vi "Set Default Word.vi"(8 "error in":errorcluster, 10 "default word":u32 format="%032b", 11 "label ref in":T1 format="%.0x") -> (0 "error out":errorcluster, 3 "label ref out":T1 format="%.0x")   [LabVIEW 2020, in "ARINC 429 Scripting.lvlib"]
uses:
  ARINC 429 Scripting.lvlib
  <vilib>/NI VeriStand/Custom Device API/Custom Device API.lvlib
  <vilib>/NI VeriStand/Custom Device API/Set Item Property (U32).vi
  AIM/Constants.vi
  AIM/AIM ARINC 429 Scripting.lvlib
  <vilib>/NI VeriStand/Custom Device API/Custom Device Item Ref.ctl
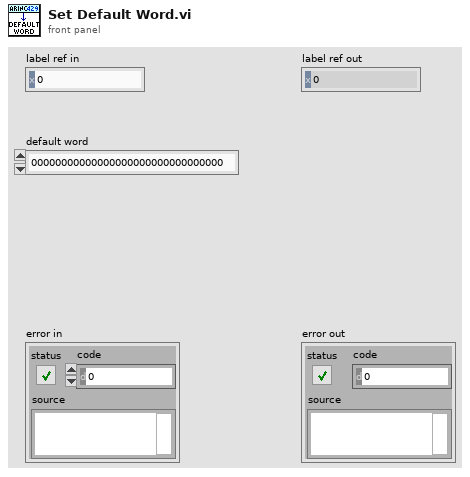
[diagram p1: front panel]
types:
  T1 = typedef "Custom Device API.lvlib/Custom Device Item Ref.ctl" = u64
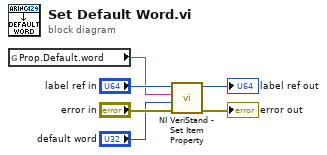
[diagram p0: block diagram]
diagram:
  n1 = global read "Constants.vi" "Prop.Default.word"() -> (w2:string)
  n2 = call-poly <vilib>:"NI VeriStand - Set Item Property.vi"("error in (no error)"="error in", "Value"="default word", "Property Name"=w2, "Item Ref in"="label ref in") -> ("error out"=→"error out":errorcluster, "Item Ref out"=→"label ref out":T1)  [unwired: 5 in, 1 out]
